vi "GetNodeCall.vi"(5 "name":string, 6 "error in":errorcluster, 9 "PythonConverter in":refnum<class "PythonBDConverter.lvclass">) -> (0 "error out":errorcluster, 3 "PythonConverter out":refnum<class "PythonBDConverter.lvclass">, 4 "call":string)   [LabVIEW 2014, in "PythonBDConverter.lvclass"]
uses:
  PythonBDConverter.lvclass
  PythonBDConverter.lvclass/PythonBDConverter.ctl
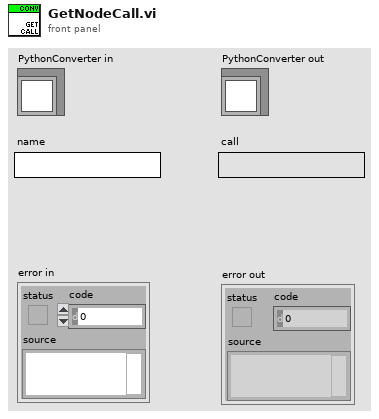
[diagram p1: front panel]
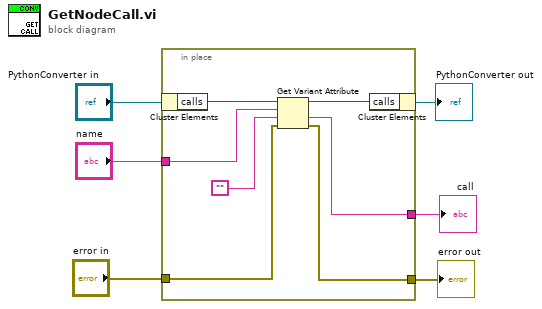
[diagram p0: block diagram]
diagram:
  n1 = in-place {
    in-place-border: "error in" -> [w11]
    in-place-border: [w10] -> w3
    in-place-border: "name" -> [w9]
    in-place-border: [w7] -> w1
    n2 = in-place-cluster #1("PythonConverter in") -> ("calls"=w13:variant)
    n3 = Get Variant Attribute(Variant=w13, name=w9, default value (empty Variant)="", error in=w11) -> (duplicate Variant=w12:variant, value=w7:string, error out=w10:errorcluster)  [unwired: 1 out]
    n4 = in-place-cluster #1("calls"=w12) -> (→"PythonConverter out":refnum<class "PythonBDConverter.lvclass">)
  }
  "error out" <- w3
  "call" <- w1
